vi "Begin.vi"(8 "error in":errorcluster) -> (0 "error out":errorcluster)   [LabVIEW 2018]
doc: "Called before other user functions, this VI can be used to open I/O refnums, load in file data, and do general program initialization. Notice that the <B>error out</B> terminal is simply used for data flow. Wiring it to other structures or subVIs ensures that this VI runs first."
uses:
  <vilib>/Rock Robotics/WPI/DriverStation/WPI_DriverStationRobotMode2.ctl
  <vilib>/Rock Robotics/WPI/Joystick/WPI_JoystickDeviceEnum.ctl
  <vilib>/Rock Robotics/WPI/Solenoid/WPI_SolenoidChannel.ctl
  <vilib>/Rock Robotics/WPI/Solenoid/WPI_SolenoidValue.ctl
  <vilib>/Rock Robotics/SystemInterfaces/DIO/FPGA_DIOPWMChannel.ctl
  <vilib>/Rock Robotics/WPI/SafetyOutput/WPI_SafetyOutputConfigMenu.ctl
  Robot Global Data.vi
  <vilib>/Rock Robotics/WPI/Solenoid/WPI_SolenoidOpenSingle.vi
  <vilib>/Rock Robotics/WPI/Solenoid/WPI_SolenoidSetEnum.vi
  <vilib>/Rock Robotics/WPI/MotorControl/WPI_MotorControlOpen SPARK.vi
  <vilib>/Rock Robotics/WPI/RobotDrive/WPI_RobotDriveOpen4MotorWithExistingMotors.vi
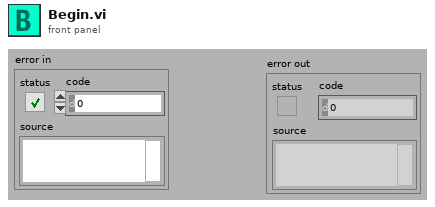
[diagram p1: front panel]
types:
  T1 = typedef "WPI_SafetyOutputConfigMenu.ctl" = enum16{"Enable", "Disable"}
  T2 = typedef "FPGA_DIOPWMChannel.ctl" = enum8{"PWM 0", "PWM 1", "PWM 2", "PWM 3", "PWM 4", "PWM 5", "PWM 6", "PWM 7", "PWM 8", "PWM 9", "PWM MXP 0", "PWM MXP 1", "PWM MXP 2", "PWM MXP 3", "PWM MXP 4", "PWM MXP 5", "PWM MXP 6", "PWM MXP 7", "PWM MXP 8", "PWM MXP 9", "Invalid"}
  T3 = typedef "WPI_SolenoidValue.ctl" = enum16{"Off", "On", "Forward", "Reverse"}
  T4 = typedef "WPI_SolenoidChannel.ctl" = enum8{"Solenoid 0", "Solenoid 1", "Solenoid 2", "Solenoid 3", "Solenoid 4", "Solenoid 5", "Solenoid 6", "Solenoid 7", "Invalid"}
  T5 = typedef "WPI_JoystickDeviceEnum.ctl" = enum16{"USB 0", "USB 1", "USB 2", "USB 3", "USB 4", "USB 5"}
  T6 = typedef "WPI_DriverStationRobotMode2.ctl" = enum16{"Autonomous Disabled", "Autonomous Enabled", "Teleop Disabled", "Teleop Enabled", "Disconnected", "Finish", "Test Disabled", "Test Enabled", "Emergency Stopped"}
  T7 = typedef "WPI_JoystickDevRef.ctl" = cluster{"Device":T5}
  T8 = typedef "WPI_MotorControlDeviceRef.ctl" = cluster{"DeviceStatus":errorcluster, "Type":T9, "PWM":cluster{"PWM Channel":T2, "DeadBand":T10}, "CAN":cluster{"Device Number":u8, "SetOutput VI Ref":variant, "GetOutput VI Ref":variant, "Enable VI Ref":variant, "Disable VI Ref":variant, "Data":variant}, "Invert":bool, "DIO PWM":cluster{"PWM \"Enable\" Channel":T2, "DIOChannel":T11, "PWM Rate":dbl}}
  T9 = typedef "WPI_MotorControlType.ctl" = enum16{"PWM", "CAN", "DIO PWM"}
  T10 = typedef "WPI_PWMDeadband.ctl" = cluster{"Name":string, "maxPositivePwm":i32, "minPositivePwm":i32, "centerPwm":i32, "maxNegativePwm":i32, "minNegativePwm":i32, "angularRange":u16}
  T11 = typedef "FPGA_DIOChannel.ctl" = enum8{"DIO 0", "DIO 1", "DIO 2", "DIO 3", "DIO 4", "DIO 5", "DIO 6", "DIO 7", "DIO 8", "DIO 9", "DIO MXP 0", "DIO MXP 1", "DIO MXP 2", "DIO MXP 3", "DIO MXP 4", "DIO MXP 5", "DIO MXP 6", "DIO MXP 7", "DIO MXP 8", "DIO MXP 9", "DIO MXP 10", "DIO MXP 11", "DIO MXP 12", "DIO MXP 13", "DIO MXP 14", "DIO MXP 15", "SPI Port CS1", "SPI Port CS2", "SPI Port CS3", "SPI Port MISO", "SPI Port MOSI", "Invalid"}
  T12 = typedef "Command Status Info.ctl" = cluster{"Name":string, "Status":T13, "notifier out":T14}
  T13 = typedef "Completion Status.ctl" = enum16{"Successful", "Aborted", "Incomplete"}
  T14 = typedef "Completion Notifier.ctl" = refnum<notifier>
  T15 = typedef "WPI_RobotDriveDevRef.ctl" = cluster{"DevStatus":errorcluster, "Motors[]":T8[], "Square Inputs":bool, "Max Output":dbl}
  T16 = typedef "WPI_SolenoidDevRef.ctl" = cluster{"DevStatus":errorcluster, "Pneumatics Control Module":u8, "Forward Solenoid Channel":T4, "Reverse Solenoid Channel":T4}
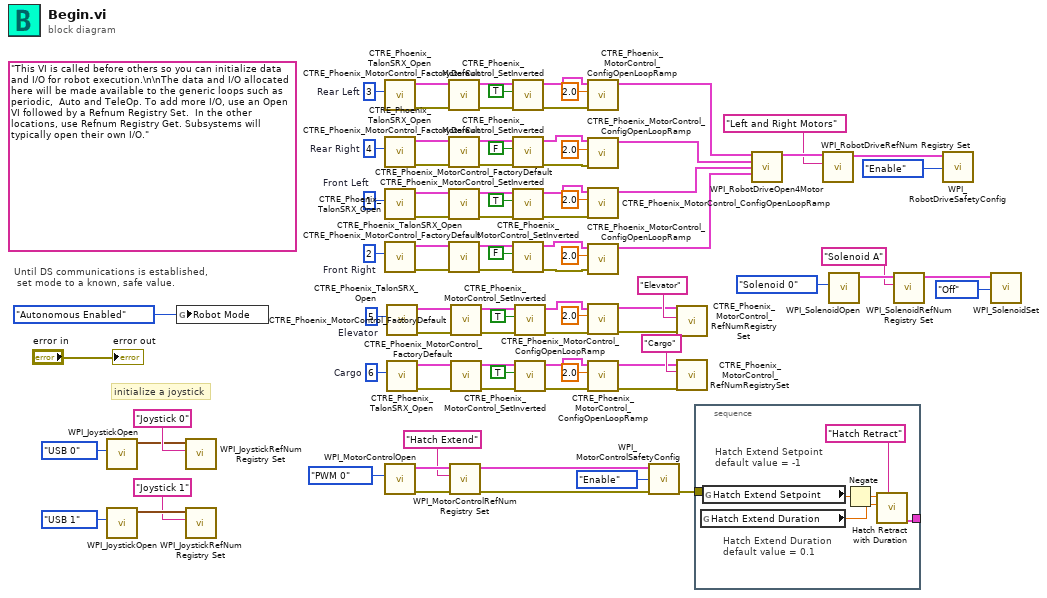
[diagram p0: block diagram]
diagram:
  w46 = u8 6  # Cargo
  w57 = u8 5  # Elevator
  w58 = u8 2  # Front Right
  w69 = u8 1  # Front Left
  w70 = u8 4  # Rear Right
  w81 = u8 3  # Rear Left
  (unwired) "This VI is called before others so you can initialize data and I/O for robot execution.\n\nThe data and I/O allocated here will be made available to the generic loops such as periodic,  Auto and TeleOp. To add more I/O, use an Open VI followed by a Refnum Registry Set.  In the other locations, use Refnum Registry Get. Subsystems will typically open their own I/O."
  # "initialize a joystick"
  # "Until DS communications is established,\n set mode to a known, safe value."
  n1 = call <vilib>:"WPI_JoystickOpen.vi"("JoystickDevice"=WPI_JoystickDeviceEnum."USB 0") -> ("JoystickDevRef"=w87:T7)  [unwired: 10 in]
  n2 = call <vilib>:"WPI_JoystickOpen.vi"("JoystickDevice"=WPI_JoystickDeviceEnum."USB 1") -> ("JoystickDevRef"=w83:T7)  [unwired: 10 in]
  n3 = global write "Robot Global Data.vi" "Robot Mode"(WPI_DriverStationRobotMode2."Autonomous Enabled" ("Robot Mode")) -> ()
  n4 = call <vilib>:"WPI_JoystickRefNum Registry Set.vi"("refnum name"="Joystick 0", "JoystickDevRef"=w87) -> ()  [unwired: 8 in, 2 out]
  n5 = call <vilib>:"WPI_JoystickRefNum Registry Set.vi"("refnum name"="Joystick 1", "JoystickDevRef"=w83) -> ()  [unwired: 8 in, 2 out]
  n6 = call <vilib>:"CTRE_Phoenix_TalonSRX_Open.vi"("Device Number"=w81) -> ("error out"=w78:errorcluster, "CAN Talon SRX Ref"=w80:T8)  [unwired: 9 in]
  n7 = call <vilib>:"CTRE_Phoenix_TalonSRX_Open.vi"("Device Number"=w70) -> ("error out"=w73:errorcluster, "CAN Talon SRX Ref"=w71:T8)  [unwired: 9 in]
  n8 = call <vilib>:"CTRE_Phoenix_TalonSRX_Open.vi"("Device Number"=w69) -> ("error out"=w66:errorcluster, "CAN Talon SRX Ref"=w68:T8)  [unwired: 9 in]
  n9 = call <vilib>:"CTRE_Phoenix_TalonSRX_Open.vi"("Device Number"=w58) -> ("error out"=w61:errorcluster, "CAN Talon SRX Ref"=w59:T8)  [unwired: 9 in]
  n10 = call-poly <vilib>:"WPI_MotorControlOpen.vi"("PWM Channel"=FPGA_DIOPWMChannel."PWM 0") -> ("error out"=w31:errorcluster, "MotorControlDeviceRef"=w33:T8)  [unwired: 9 in]
  n11 = call <vilib>:"CTRE_Phoenix_TalonSRX_Open.vi"("Device Number"=w57) -> ("error out"=w54:errorcluster, "CAN Talon SRX Ref"=w56:T8)  [unwired: 9 in]
  n12 = call <vilib>:"CTRE_Phoenix_TalonSRX_Open.vi"("Device Number"=w46) -> ("error out"=w49:errorcluster, "CAN Talon SRX Ref"=w47:T8)  [unwired: 9 in]
  n13 = call <vilib>:"CTRE_Phoenix_MotorControl_FactoryDefault.vi"("error in"=w78, "PhoenixMotorControlDevRef"=w80) -> ("error out"=w77:errorcluster, "PhoenixMotorControlDevRef"=w79:T8)  [unwired: 8 in]
  n14 = call <vilib>:"CTRE_Phoenix_MotorControl_FactoryDefault.vi"("error in"=w73, "PhoenixMotorControlDevRef"=w71) -> ("error out"=w74:errorcluster, "PhoenixMotorControlDevRef"=w72:T8)  [unwired: 8 in]
  n15 = call <vilib>:"CTRE_Phoenix_MotorControl_FactoryDefault.vi"("error in"=w66, "PhoenixMotorControlDevRef"=w68) -> ("error out"=w65:errorcluster, "PhoenixMotorControlDevRef"=w67:T8)  [unwired: 8 in]
  n16 = call <vilib>:"CTRE_Phoenix_MotorControl_FactoryDefault.vi"("error in"=w61, "PhoenixMotorControlDevRef"=w59) -> ("error out"=w62:errorcluster, "PhoenixMotorControlDevRef"=w60:T8)  [unwired: 8 in]
  n17 = call <vilib>:"WPI_MotorControlRefNum Registry Set.vi"("error in (no error)"=w31, "refnum name"="Hatch Extend", "MotorControlDevRef"=w33) -> ("error out"=w29:errorcluster, "MotorControlDevRef"=w32:T8)  [unwired: 7 in]
  n18 = call <vilib>:"CTRE_Phoenix_MotorControl_FactoryDefault.vi"("error in"=w54, "PhoenixMotorControlDevRef"=w56) -> ("error out"=w53:errorcluster, "PhoenixMotorControlDevRef"=w55:T8)  [unwired: 8 in]
  n19 = call <vilib>:"CTRE_Phoenix_MotorControl_FactoryDefault.vi"("error in"=w49, "PhoenixMotorControlDevRef"=w47) -> ("error out"=w50:errorcluster, "PhoenixMotorControlDevRef"=w48:T8)  [unwired: 8 in]
  n20 = call <vilib>:"CTRE_Phoenix_MotorControl_SetInverted.vi"("error in (no error)"=w77, "Invert?"=TRUE, "PhoenixMotorControlDevRef"=w79) -> ("error out"=w20:errorcluster, "PhoenixMotorControlDevRef"=w9:T8)  [unwired: 7 in]
  n21 = call <vilib>:"CTRE_Phoenix_MotorControl_SetInverted.vi"("error in (no error)"=w74, "Invert?"=FALSE, "PhoenixMotorControlDevRef"=w72) -> ("error out"=w19:errorcluster, "PhoenixMotorControlDevRef"=w10:T8)  [unwired: 7 in]
  n22 = call <vilib>:"CTRE_Phoenix_MotorControl_SetInverted.vi"("error in (no error)"=w65, "Invert?"=TRUE, "PhoenixMotorControlDevRef"=w67) -> ("error out"=w18:errorcluster, "PhoenixMotorControlDevRef"=w11:T8)  [unwired: 7 in]
  n23 = call <vilib>:"CTRE_Phoenix_MotorControl_SetInverted.vi"("error in (no error)"=w62, "Invert?"=FALSE, "PhoenixMotorControlDevRef"=w60) -> ("error out"=w17:errorcluster, "PhoenixMotorControlDevRef"=w12:T8)  [unwired: 7 in]
  n24 = call <vilib>:"CTRE_Phoenix_MotorControl_SetInverted.vi"("error in (no error)"=w53, "Invert?"=TRUE, "PhoenixMotorControlDevRef"=w55) -> ("error out"=w16:errorcluster, "PhoenixMotorControlDevRef"=w13:T8)  [unwired: 7 in]
  n25 = call <vilib>:"CTRE_Phoenix_MotorControl_SetInverted.vi"("error in (no error)"=w50, "Invert?"=TRUE, "PhoenixMotorControlDevRef"=w48) -> ("error out"=w15:errorcluster, "PhoenixMotorControlDevRef"=w14:T8)  [unwired: 7 in]
  n26 = call <vilib>:"CTRE_Phoenix_MotorControl_ConfigOpenLoopRamp.vi"("error in (no error)"=w20, "secondsFromNeutralToFull"=2.0, "PhoenixMotorControlDevRef"=w9) -> ("PhoenixMotorControlDevRef"=w8:T8)  [unwired: 7 in, 1 out]
  n27 = call <vilib>:"CTRE_Phoenix_MotorControl_ConfigOpenLoopRamp.vi"("error in (no error)"=w19, "secondsFromNeutralToFull"=2.0, "PhoenixMotorControlDevRef"=w10) -> ("PhoenixMotorControlDevRef"=w7:T8)  [unwired: 7 in, 1 out]
  n28 = call <vilib>:"CTRE_Phoenix_MotorControl_ConfigOpenLoopRamp.vi"("error in (no error)"=w18, "secondsFromNeutralToFull"=2.0, "PhoenixMotorControlDevRef"=w11) -> ("PhoenixMotorControlDevRef"=w6:T8)  [unwired: 7 in, 1 out]
  n29 = call <vilib>:"CTRE_Phoenix_MotorControl_ConfigOpenLoopRamp.vi"("error in (no error)"=w17, "secondsFromNeutralToFull"=2.0, "PhoenixMotorControlDevRef"=w12) -> ("PhoenixMotorControlDevRef"=w5:T8)  [unwired: 7 in, 1 out]
  n30 = call <vilib>:"CTRE_Phoenix_MotorControl_ConfigOpenLoopRamp.vi"("error in (no error)"=w16, "secondsFromNeutralToFull"=2.0, "PhoenixMotorControlDevRef"=w13) -> ("error out"=w3:errorcluster, "PhoenixMotorControlDevRef"=w4:T8)  [unwired: 7 in]
  n31 = call <vilib>:"CTRE_Phoenix_MotorControl_ConfigOpenLoopRamp.vi"("error in (no error)"=w15, "secondsFromNeutralToFull"=2.0, "PhoenixMotorControlDevRef"=w14) -> ("error out"=w1:errorcluster, "PhoenixMotorControlDevRef"=w2:T8)  [unwired: 7 in]
  n32 = call <vilib>:"WPI_MotorControlSafetyConfig.vi"("error in (no error)"=w29, "mode"=WPI_SafetyOutputConfigMenu."Enable", "MotorControlDevRef"=w32) -> ("error out"=w27:errorcluster)  [unwired: 7 in, 1 out]
  n33 = call <vilib>:"CTRE_Phoenix_MotorControl_RefNumRegistrySet.vi"("error in (no error)"=w3, "refnum name"="Elevator", "PhoenixMotorControlDevRef"=w4) -> ()  [unwired: 7 in, 2 out]
  n34 = call <vilib>:"CTRE_Phoenix_MotorControl_RefNumRegistrySet.vi"("error in (no error)"=w1, "refnum name"="Cargo", "PhoenixMotorControlDevRef"=w2) -> ()  [unwired: 7 in, 2 out]
  n35 = stacked-sequence {
    tunnel: [w94] -> _
    tunnel: w27 -> [_]
    frame #0 {
      # "Hatch Extend Setpoint\ndefault value = -1"
      # "Hatch Extend Duration\ndefault value = 0.1"
      n36 = global read "Robot Global Data.vi" "Hatch Extend Duration"() -> (w92:dbl)
      n37 = global read "Robot Global Data.vi" "Hatch Extend Setpoint"() -> (w93:dbl)
      n38 = Negate(x=w93) -> (-x=w91:dbl)
      n39 = call "Hatch Retract with Duration.vi"("Description"="Hatch Retract", "Duration (s)"=w92, "Setpoint"=w91) -> ("Command Info Out"=w94:T12)  [unwired: 8 in]
    }
  }
  n40 = call-poly <vilib>:"WPI_RobotDriveOpen4Motor.vi"("Rear Left Motor Dev Ref"=w8, "Rear Right Motor Dev Ref"=w7, "Front Left Motor Dev Ref"=w6, "Front Right Motor Dev Ref"=w5) -> ("RobotDriveDevRef"=w45:T15)  [unwired: 10 in, 1 out]
  n41 = call <vilib>:"WPI_RobotDriveRefNum Registry Set.vi"("refnum name"="Left and Right Motors", "RobotDriveDevRef"=w45) -> ("RobotDriveDevRef"=w44:T15)  [unwired: 8 in, 1 out]
  n42 = call-poly <vilib>:"WPI_SolenoidOpen.vi"("Solenoid Channel"=WPI_SolenoidChannel."Solenoid 0") -> ("SolenoidDevRef"=w38:T16)  [unwired: 9 in, 1 out]
  n43 = call <vilib>:"WPI_SolenoidRefNum Registry Set.vi"("refnum name"="Solenoid A", "SolenoidDevRef"=w38) -> ("SolenoidDevRef"=w37:T16)  [unwired: 8 in, 1 out]
  n44 = call <vilib>:"WPI_RobotDriveSafetyConfig.vi"("mode"=WPI_SafetyOutputConfigMenu."Enable", "RobotDriveDevRef"=w44) -> ()  [unwired: 8 in, 2 out]
  n45 = call-poly <vilib>:"WPI_SolenoidSet.vi"("Value"=WPI_SolenoidValue."Off", "SolenoidDevRef"=w37) -> ()  [unwired: 8 in, 2 out]
  "error out" <- "error in"
